vi "Utility.GetDUTIndex.vi"(9 "DUTs":string[](array[string]), 11 "Channel":string) -> (2 "Found?":bool, 3 "Index":i32)   [LabVIEW 2014, in "NIAnalysis.lvlib"]
uses:
  NIAnalysis.lvlib
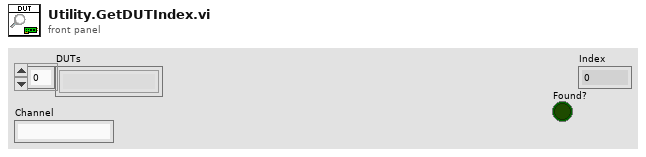
[diagram p1: front panel]
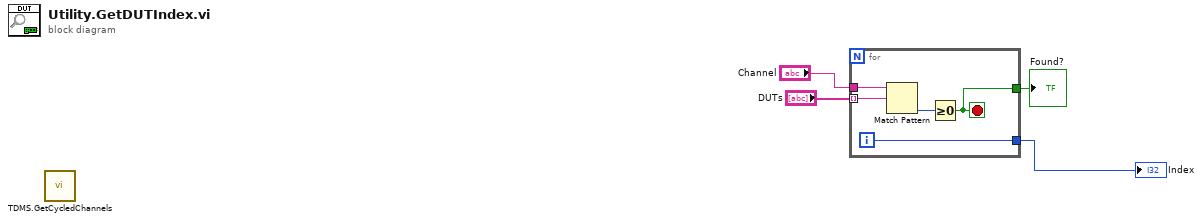
[diagram p0: block diagram]
diagram:
  n1 = call "TDMS.GetCycledChannels.vi"() -> ()  [unwired: 8 in, 4 out]
  n2 = for {
    tunnel: "Channel" -> [w9]
    tunnel: [w7] -> w3
    tunnel: [w6] -> w2
    tunnel: "DUTs" -> [w5] mode=indexing
    i -> [w7]
    stop <- w6 stop-if-true
    n3 = Match Pattern(string=w9, regular expression=w5) -> (offset past match=w8:i32)  [unwired: 1 in, 3 out]
    n4 = Greater Or Equal To 0?(x=w8) -> (x >= 0?=w6:bool)
  }
  "Index" <- w3
  "Found?" <- w2
